vi "ExcelCreateReport.vi"(2 "error in (no error)":errorcluster, 3 "ReportSelection":u16, 4 "Input":T1, 5 "closing behavior":T2(ring)) -> (0 "error out":errorcluster, 1 "ReportPath":path)   [LabVIEW 2013, in "main.lvlib"]
uses:
  main.lvlib
  Controls/Enum Variables.ctl
  Globals/DataPathGlobalVariable.vi
  <userlib>/_OpenG.lib/file/file.llb/File Exists - Scalar__ogtk.vi
  <userlib>/Excel/excel.llb/excel open (path).vi
  <vilib>/regexp/Match Regular Expression.xnode
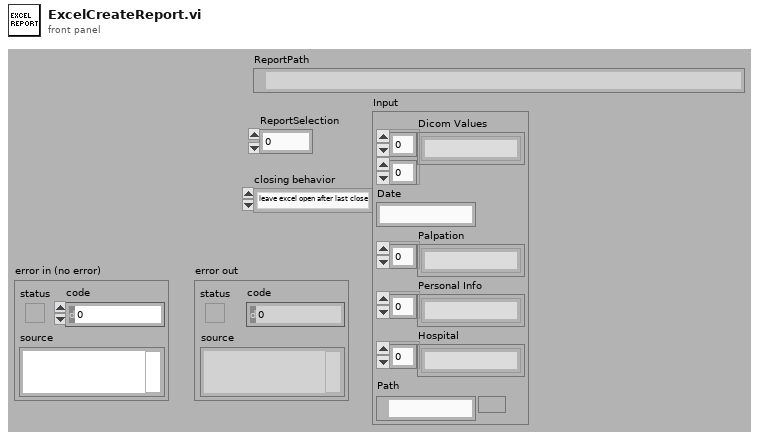
[diagram p1: front panel]
types:
  T1 = cluster{"Dicom Values":string[][], "Date":string, "Palpation":string[], "Personal Info":string[], "Hospital":string[], "Path":path}
  T2 = enum16{"leave excel open after last close", "close only if opened by LabVIEW", "close excel after last close"}
  T3 = typedef "main.lvlib/Enum Variables.ctl" = enum16{"SetAcqFilter", "GetAcqFilter", "Set Filter", "Get Filter", "Set Height", "Get Height", "Set Recorded Height", "Get Recorded Height", "Set Blue Pressure", "Get Blue Pressure", "Set Red Pressure", "Get Red Pressure", "Init", "Reset Pressure", "Set Red Cursors", "Get Red Cursors", "Set Blue Cursors", "Get Blue Cursors", "Set Language", "Get Language", "Set Active Graphs", "Get ActiveGraphs", "Set Method", "Get Method", "Set Encryption", "Get Encryption", "Set ExcelVersion", "Get ExcelVersion", "Set DICOM Avail", "Get DICOM Avail", "Set DICOM Encode", "Get DICOM Encode", "Set JournalExport", "Get JournalExport", "Set Sequence", "Get Sequence", "Set DAQ Connected", "Get DAQ Connected", "Set Current Graph", "Get Current Graph", "Set General Settings", "Get Hyphenation", "Set Arm Calc Method", "Get Arm Calc Method", "Set Dicom Tags", "Get Dicom Tags", "Set BT Serial", "Get BT Serial", "Set BT Accepted Serials", "Get BT Accepted Serials", "Get BT License", "Set BT License"}
  T4 = enum16{"open workbook as template", "open workbook from file", "create new workbook"}
  T5 = typedef "excel Object Reference.ctl" = refnum<k1>
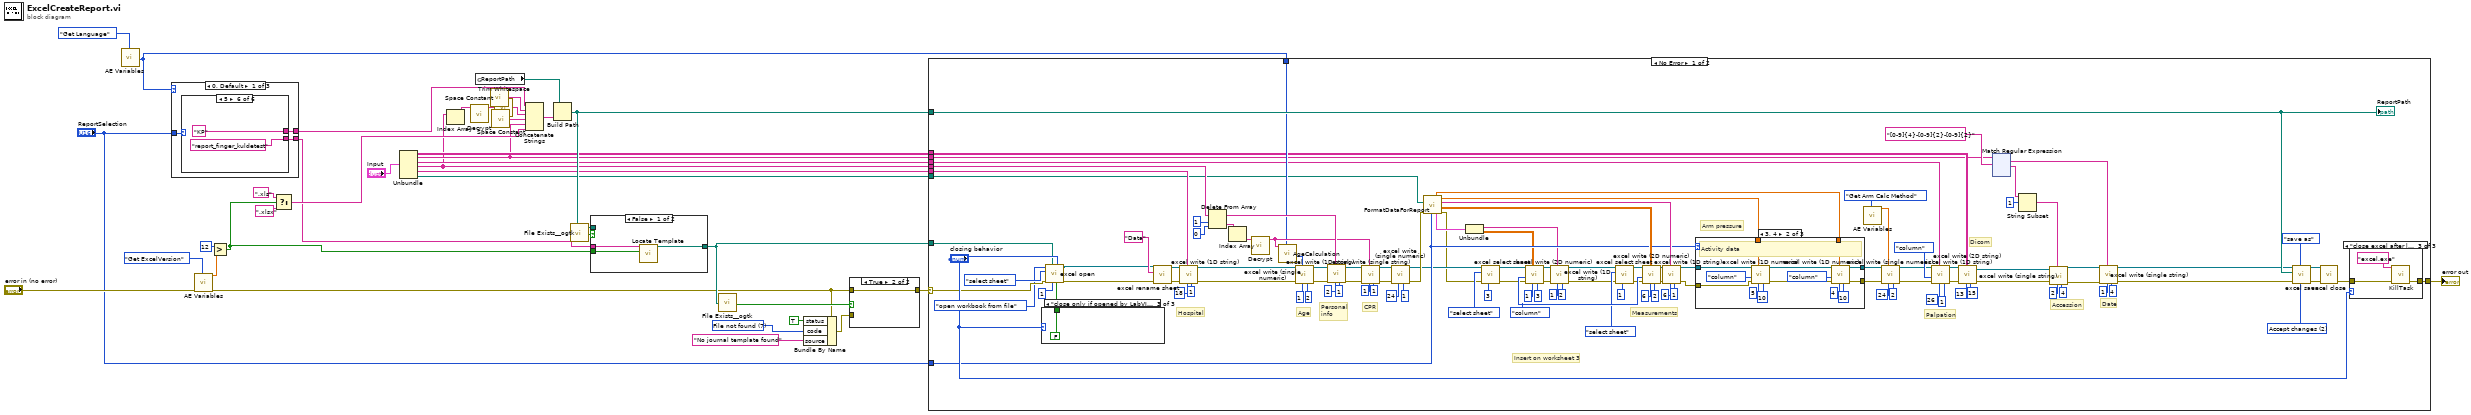
[diagram p0: block diagram]
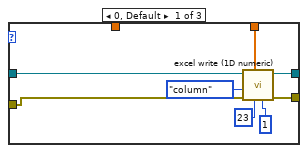
[diagram p2: hidden frame]
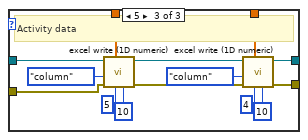
[diagram p3: hidden frame]
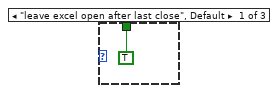
[diagram p6: hidden frame]
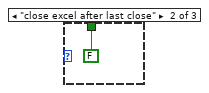
[diagram p7: hidden frame]
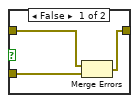
[diagram p9: hidden frame]
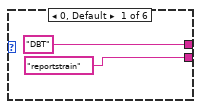
[diagram p10: hidden frame]
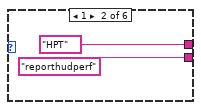
[diagram p11: hidden frame]
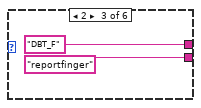
[diagram p12: hidden frame]
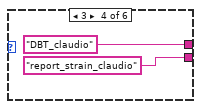
[diagram p13: hidden frame]
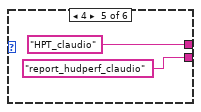
[diagram p14: hidden frame]
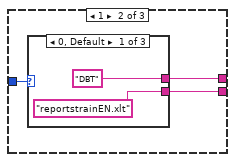
[diagram p15: hidden frame]
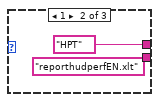
[diagram p16: hidden frame]
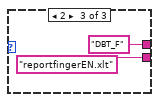
[diagram p17: hidden frame]
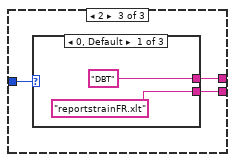
[diagram p18: hidden frame]
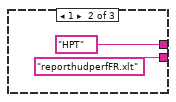
[diagram p19: hidden frame]
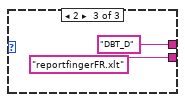
[diagram p20: hidden frame]
diagram:
  w8 = 7 items=["No error", "Argument error", "Memory is full", "Out of zone", "End of file", "File already open", "Generic file I/O error", "File not found", "File permission error", "Disk is full", "Duplicate path", "Too many files open", "System feature not enabled", "Resource file not found", "Cannot add resource", "Resource not found", "Image not found", "Image memory error", "Pen does not exist", "Config type invalid", "Config token not found", "Config parse error", "Config memory error", "Bad external code format", "Bad external code offset", "External code not present", "Null window", "Destroy window error", "Null menu", "Print aborted", "Bad print record", "Print driver error", "Windows error during printing", "Memory error during printing", "Print dialog error", "Generic print error", "Invalid device refnum", "Device not found", "Device parameter error", "Device unit error", "Cannot open device", "Device call aborted", "Generic error", "Cancelled by user", "Object ID too low", "Object ID too high", "Object not in heap", "Unknown heap", "Unknown object (invalid DefProc)", "Unknown object (DefProc not in table)", "Message out of range", "Invalid (null) method", "Unknown message", "Manager call not supported", "Bad address", "Network operation in progress", "Network operation timed out", "Connection is busy", "Network attribute not supported", "Network error", "Address in use", "System out of memory", "Connection aborted", "Connection refused", "Not connected", "Already connected", "Connection closed", "Initialization error (interapplication manager)", "Bad occurrence", "Wait on unbound occurrence handler", "Occurrence queue overflow", "Datalog type conflict", "Unused", "Unrecognized type (interapplication manager)", "Memory corrupt", "Failed to make temporary DLL", "Old CIN version", "Drag socket not found", "Failed to load drop-object", "Failed to register OLE object", "Failed to release OLE object", "Format specifier type mismatch", "Unknown format specifier", "Too few format specifiers", "Too many format specifiers", "Scan failed", "Newer CIN version", "Error converting to variant", "Runtime menu error", "Password tampered", "Variant attribute not found", "Incompatible variant data type", "Event data is not available", "Event Store is not present", "Occurrence is not found", "Event Queue is not created", "Event info is not available", "Refnum passed is NULL", "Error retrieving Class GUID", "Error retrieving CoClass GUID", "Error retrieving TypeLib GUID.", "Bad built application magic bytes.", "Specific driver is different from the specific driver associated with the Logical Name.", "There is no session opened to the class driver.", "Max Error", "MAX - Error with config objects", "MAX - Error loading configuration", "MAX - Group not supported"]
  n1 = call "AE Variables.vi"("Action"=Enum_Variables."Get Language") -> ("RingOut"=w19:u16)  [unwired: 11 in, 7 out]
  n2 = case shown="0, Default" w19 {
    tunnel: [w41 w56 w65] -> w2
    tunnel: "ReportSelection" -> [w40 w55 w64]
    tunnel: [w39 w54 w63] -> w36
    frame 0, Default {
      n3 = case shown="5" w40 {
        tunnel: ["reportstrain" "reporthudperf" "reportfinger" "report_strain_claudio" "report_hudperf_claudio" "report_finger_kuldetest"] -> w41
        tunnel: ["DBT" "HPT" "DBT_F" "DBT_claudio" "HPT_claudio" "KP"] -> w39
        frame 0, Default {
        }
        frame 1 {
        }
        frame 2 {
        }
        frame 3 {
        }
        frame 4 {
        }
        frame 5 {
        }
      }
    }
    frame 1 {
      n4 = case shown="0, Default" w55 {
        tunnel: ["reportstrainEN.xlt" "reporthudperfEN.xlt" "reportfingerEN.xlt"] -> w56
        tunnel: ["DBT" "HPT" "DBT_F"] -> w54
        frame 0, Default {
        }
        frame 1 {
        }
        frame 2 {
        }
      }
    }
    frame 2 {
      n5 = case shown="0, Default" w64 {
        tunnel: ["reportstrainFR.xlt" "reporthudperfFR.xlt" "reportfingerFR.xlt"] -> w65
        tunnel: ["DBT" "HPT" "DBT_D"] -> w63
        frame 0, Default {
        }
        frame 1 {
        }
        frame 2 {
        }
      }
    }
  }
  n6 = call "AE Variables.vi"("error in (no error)"="error in (no error)", "Action"=Enum_Variables."Get ExcelVersion") -> ("NumericOut"=w22:dbl, "error out"=w9:errorcluster)  [unwired: 10 in, 6 out]
  n7 = Greater?(x=12, y=w22) -> (0:w1:bool)
  n8 = Select(t=".xls", s=w1, f=".xlsx") -> (s? t:f=w27:string)
  n9 = Unbundle("Input") -> ("Dicom Values"=w15:string[][], "Date"=w6:string, "Palpation"=w18:string[], "Personal Info"=w4:string[], "Hospital"=w17:string[], "Path"=w16:path)
  n10 = Index Array(array=w4) -> (element=w34:string)  [unwired: 1 in]
  n11 = call "Decrypt.vi"("Input"=w34) -> ("Output"=w32:string)  [unwired: 10 in]
  n12 = global read "DataPathGlobalVariable.vi" "ReportPath"() -> (w38:path)
  n13 = call <vilib>:"Space Constant.vi"() -> ("String"=w35:string)
  n14 = call <vilib>:"Space Constant.vi"() -> ("String"=w37:string)
  n15 = call <vilib>:"Trim Whitespace.vi"("string"=w32) -> ("trimmed string"=w31:string)  [unwired: 1 in]
  n16 = Concatenate Strings(w36, w35, w31, w37, w6, w27) -> (w33:string)
  n17 = Build Path(base path=w38, name or relative path=w33) -> (appended path=w25:path)
  n18 = call-poly <userlib>:"File Exists__ogtk.vi"("file path"=w25) -> ("exists"=w26:bool)  [unwired: 6 in, 1 out]
  n19 = case shown="False" w26 {
    tunnel: w2 -> [w74 _]
    tunnel: [w72 w75] -> w14
    tunnel: w25 -> [_ w75]
    tunnel: w1 -> [w73 _]
    frame False {
      n20 = call "Locate Template.vi"("Old excel"=w73, "File name"=w74) -> ("Path"=w72:path)  [unwired: 9 in]
    }
    frame True {
    }
  }
  n21 = call-poly <userlib>:"File Exists__ogtk.vi"("file path"=w14) -> ("exists"=w13:bool)  [unwired: 6 in, 1 out]
  n22 = Bundle By Name(cluster=w9, "status"=TRUE, "code"=w8, "source"="No journal template found") -> (w11:errorcluster)
  n23 = case shown="True" w13 {
    tunnel: w9 -> [w78 w79]
    tunnel: [w77 w79] -> w7
    tunnel: w11 -> [w76 _]
    frame False {
      n24 = Merge Errors(w78, w76) -> (w77:errorcluster)
    }
    frame True {
    }
  }
  n25 = case shown="No Error" w7 {
    selector: w7 -> [w157 w352]
    tunnel: [w155 w352] -> w30
    tunnel: w25 -> [w165 _]
    tunnel: w19 -> [w162 _]
    tunnel: w18 -> [w152 _]
    tunnel: w4 -> [w145 _]
    tunnel: w17 -> [w146 _]
    tunnel: w16 -> [w144 _]
    tunnel: w15 -> [w161 _]
    tunnel: w14 -> [w158 _]
    tunnel: w6 -> [w92 _]
    tunnel: "ReportSelection" -> [w124 _]
    frame No Error {
      w106 = enum16{"row", "column"}."column" ("Write array by (row)")
      w181 = u16 2 items=["Prompt for changes"=1, "Accept changes"=2, "Reject changes"=3] ("Save As options")
      # "Accession"
      # "Insert on worksheet 3"
      # "Measurements"
      # "Arm pressure"
      # "Date"
      # "Dicom"
      # "Palpation"
      # "CPR"
      # "Hospital"
      # "Personal\ninfo"
      # "Age"
      n26 = case shown="\"close only if opened by LabVIEW\"" "closing behavior" {
        tunnel: [TRUE FALSE FALSE] -> w166
        frame "leave excel open after last close", Default {
        }
        frame "close excel after last close" {
        }
        frame "close only if opened by LabVIEW" {
        }
      }
      n27 = call-poly <userlib>:"excel open.vi"("Visible (T)"=w166, "closing behavior (leave open)"="closing behavior", "worksheet_number"=u8 1, "workbook path"=w158, "error in (no error)"=w157, "select/new"=enum16{"new sheet", "select sheet"}."select sheet", "create/open template/open file"=T4."open workbook from file") -> ("error out"=w114:errorcluster, "reference"=w115:T5)  [unwired: 3 in]
      n28 = call <userlib>:"excel rename sheet.vi"("error in (no error)"=w114, "new name"="Data", "reference"=w115) -> ("error out"=w119:errorcluster, "duplicate reference"=w120:T5)  [unwired: 5 in, 2 out]
      n29 = call <userlib>:"excel write (1D string).vi"("Column"=u32 1, "Row"=u32 18, "1D string array"=w146, "error in (no error)"=w119, "reference"=w120) -> ("error out"=w185:errorcluster, "duplicate reference"=w184:T5)  [unwired: 5 in]
      n30 = Delete From Array(array=w145, length=1, index=0) -> (deleted portion=w169:string[], array with subset deleted=w180:string[])
      n31 = Index Array(array=w169) -> (element=w168:string)  [unwired: 1 in]
      n32 = call "Decrypt.vi"("Input"=w168) -> ("Output"=w163:string)  [unwired: 10 in]
      n33 = call "AgeCalculation.vi"("Language"=w162, "CPR"=w163) -> ("Age"=w164:i32)  [unwired: 9 in]
      n34 = call <userlib>:"excel write (single numeric).vi"("Column"=u32 2, "Row"=u32 1, "Numeric"=w164, "error in (no error)"=w185, "reference"=w184) -> ("error out"=w172:errorcluster, "duplicate reference"=w173:T5)  [unwired: 5 in]
      n35 = call <userlib>:"excel write (1D string).vi"("Column"=u32 1, "Row"=u32 2, "1D string array"=w180, "error in (no error)"=w172, "reference"=w173) -> ("error out"=w174:errorcluster, "duplicate reference"=w175:T5)  [unwired: 5 in]
      n36 = call <userlib>:"excel write (single string).vi"("Column"=u32 1, "Row"=u32 1, "String"=w163, "error in (no error)"=w174, "reference"=w175) -> ("error out"=w176:errorcluster, "duplicate reference"=w177:T5)  [unwired: 5 in]
      n37 = call <userlib>:"excel write (single numeric).vi"("Column"=u32 1, "Row"=u32 24, "error in (no error)"=w176, "reference"=w177) -> ("error out"=w126:errorcluster, "duplicate reference"=w84:T5)  [unwired: 6 in]
      n38 = call "FormatDataForReport.vi"("Report selection"=w124, "error in (no error)"=w126, "Path"=w144) -> ("error out"=w83:errorcluster, "Data"=w127:dbl[][], "Names"=w128:string[], "Activity armpressure"=w122:dbl[], "output cluster"=w113:cluster{"Names":string[], "Data":dbl[][]}, "Normal armpressure"=w121:dbl[])  [unwired: 3 in]
      n39 = Unbundle(w113) -> ("Names"=w105:string[], "Data"=w104:dbl[][])
      n40 = call <userlib>:"excel select sheet.vi"("worksheet_number"=u8 3, "error in (no error)"=w83, "select/new"=enum16{"new sheet", "select sheet"}."select sheet", "reference"=w84) -> ("error out"=w95:errorcluster, "duplicate reference"=w94:T5)  [unwired: 4 in, 2 out]
      n41 = call <userlib>:"excel write (2D numeric).vi"("Column"=u32 3, "Row"=u32 1, "2D nurmeric array"=w104, "error in (no error)"=w95, "Write array by (row)"=w106, "reference"=w94) -> ("error out"=w109:errorcluster, "duplicate reference"=w112:T5)  [unwired: 4 in]
      n42 = call <userlib>:"excel write (1D string).vi"("Column"=u32 2, "Row"=u32 1, "1D string array"=w105, "error in (no error)"=w109, "reference"=w112) -> ("error out"=w98:errorcluster, "duplicate reference"=w101:T5)  [unwired: 5 in]
      n43 = call <userlib>:"excel select sheet.vi"("worksheet_number"=u8 1, "error in (no error)"=w98, "select/new"=enum16{"new sheet", "select sheet"}."select sheet", "reference"=w101) -> ("error out"=w99:errorcluster, "duplicate reference"=w100:T5)  [unwired: 4 in, 2 out]
      n44 = call <userlib>:"excel write (2D numeric).vi"("Column"=u32 2, "Row"=u32 6, "2D nurmeric array"=w127, "error in (no error)"=w99, "Write array by (row)"=w106, "reference"=w100) -> ("error out"=w133:errorcluster, "duplicate reference"=w136:T5)  [unwired: 4 in]
      n45 = call <userlib>:"excel write (1D string).vi"("Column"=u32 1, "Row"=u32 6, "1D string array"=w128, "error in (no error)"=w133, "reference"=w136) -> ("error out"=w140:errorcluster, "duplicate reference"=w139:T5)  [unwired: 5 in]
      n46 = case shown="3, 4" w124 {
        tunnel: w139 -> [w310 w326 w340]
        tunnel: [w311 w319 w333] -> w141
        tunnel: w140 -> [w309 w325 w339]
        tunnel: w122 -> [_ w324 w338]
        tunnel: [w312 w320 w334] -> w142
        tunnel: w121 -> [w308 w316 w330]
        frame 0, Default {
          n47 = call <userlib>:"excel write (1D numeric).vi"("Column"=u32 1, "Row"=u32 23, "1D Numeric Array"=w308, "error in (no error)"=w309, "Write array by (row)"=enum16{"row", "column"}."column", "reference"=w310) -> ("error out"=w311:errorcluster, "duplicate reference"=w312:T5)  [unwired: 4 in]
        }
        frame 3, 4 {
          # "Activity data"
          n48 = call <userlib>:"excel write (1D numeric).vi"("Column"=u32 10, "Row"=u32 5, "1D Numeric Array"=w324, "error in (no error)"=w325, "Write array by (row)"=enum16{"row", "column"}."column", "reference"=w326) -> ("error out"=w318:errorcluster, "duplicate reference"=w317:T5)  [unwired: 4 in]
          n49 = call <userlib>:"excel write (1D numeric).vi"("Column"=u32 10, "Row"=u32 4, "1D Numeric Array"=w316, "error in (no error)"=w318, "Write array by (row)"=enum16{"row", "column"}."column", "reference"=w317) -> ("error out"=w319:errorcluster, "duplicate reference"=w320:T5)  [unwired: 4 in]
        }
        frame 5 {
          # "Activity data"
          n50 = call <userlib>:"excel write (1D numeric).vi"("Column"=u32 10, "Row"=u32 5, "1D Numeric Array"=w338, "error in (no error)"=w339, "Write array by (row)"=enum16{"row", "column"}."column", "reference"=w340) -> ("error out"=w332:errorcluster, "duplicate reference"=w331:T5)  [unwired: 4 in]
          n51 = call <userlib>:"excel write (1D numeric).vi"("Column"=u32 10, "Row"=u32 4, "1D Numeric Array"=w330, "error in (no error)"=w332, "Write array by (row)"=enum16{"row", "column"}."column", "reference"=w331) -> ("error out"=w333:errorcluster, "duplicate reference"=w334:T5)  [unwired: 4 in]
        }
      }
      n52 = call "AE Variables.vi"("Action"=Enum_Variables."Get Arm Calc Method") -> ("NumericOut"=w138:dbl)  [unwired: 11 in, 7 out]
      n53 = call <userlib>:"excel write (single numeric).vi"("Column"=u32 2, "Row"=u32 24, "Numeric"=w138, "error in (no error)"=w141, "reference"=w142) -> ("error out"=w123:errorcluster, "duplicate reference"=w125:T5)  [unwired: 5 in]
      n54 = call <userlib>:"excel write (1D string).vi"("Column"=u32 1, "Row"=u32 26, "1D string array"=w152, "error in (no error)"=w123, "Write array by (row)"=enum16{"row", "column"}."column", "reference"=w125) -> ("error out"=w150:errorcluster, "duplicate reference"=w151:T5)  [unwired: 4 in]
      n55 = call <userlib>:"excel write (2D string).vi"("Column"=u32 15, "Row"=u32 13, "2D string array"=w161, "error in (no error)"=w150, "reference"=w151) -> ("error out"=w87:errorcluster, "duplicate reference"=w88:T5)  [unwired: 5 in]
      n56 = xnode "Match Regular Expression"("input string"=w92, "regular expression"="[0-9]{4}-[0-9]{2}-[0-9]{2}") -> ("whole match"=w91:string, "after match"=w82:string)  [unwired: 4 in, 3 out]
      n57 = String Subset(string=w82, offset (0)=1) -> (substring=w80:string)  [unwired: 1 in]
      n58 = call <userlib>:"excel write (single string).vi"("Column"=u32 4, "Row"=u32 2, "String"=w80, "error in (no error)"=w87, "reference"=w88) -> ("error out"=w86:errorcluster, "duplicate reference"=w85:T5)  [unwired: 5 in]
      n59 = call <userlib>:"excel write (single string).vi"("Column"=u32 4, "Row"=u32 1, "String"=w91, "error in (no error)"=w86, "reference"=w85) -> ("error out"=w116:errorcluster, "duplicate reference"=w117:T5)  [unwired: 5 in]
      n60 = call <userlib>:"excel save.vi"("Save As options"=w181, "mode (save)"=enum16{"save", "save as", "save a copy as"}."save as", "error in (no error)"=w116, "Path"=w165, "reference"=w117) -> ("error out"=w192:errorcluster, "duplicate reference"=w193:T5)  [unwired: 5 in]
      n61 = call <userlib>:"excel close.vi"("error in (no error)"=w192, "reference"=w193) -> ("error out"=w156:errorcluster)  [unwired: 9 in]
      n62 = case shown="\"close excel after last close\"" "closing behavior" {
        tunnel: w156 -> [w344 w345 w346]
        tunnel: [w344 w345 w347] -> w155
        frame "leave excel open after last close", Default {
        }
        frame "close only if opened by LabVIEW" {
        }
        frame "close excel after last close" {
          n63 = call "KillTask.vi"("error in (no error)"=w346, "Taskname"="excel.exe") -> ("error out"=w347:errorcluster)  [unwired: 9 in]
        }
      }
      "ReportPath" <- w165
    }
    frame Error {
    }
  }
  "error out" <- w30
